vi "SHA-1 Test.vi"() -> ()   [LabVIEW 2021, in "WebSockets.lvlib" / "WebSocket.lvclass"]
doc: "WebSockets 2.0.1.40\nSam Sharp - MediaMongrels Ltd\nCopyright (c) 2019, MediaMongrels Ltd"
uses:
  WebSocket/WebSocket.lvclass
panel:
  out "SHA1 Data":u8[](array[numeric])=[0, 0, 0, 244, 146, 20, 24, 169, 106, 74, 162, 189, 106, 208, 220, 75, 21, 127, 121, 135] format="%.0x"
  in  "String":string
  # "SHA1(\"\")\n = da39a3ee 5e6b4b0d 3255bfef 95601890 afd80709"
  # "SHA1(\"The quick brown fox jumps over the lazy dog\") \n = 2fd4e1c6 7a2d28fc ed849ee1 bb76e739 1b93eb12"
  # "minor change - dog -> cog (notice large change, aka avalache effect, in digest)"
  # "SHA1(\"The quick brown fox jumps over the lazy cog\") \n = de9f2c7f d25e1b3a fad3e85a 0bd17d9b 100db4b3"
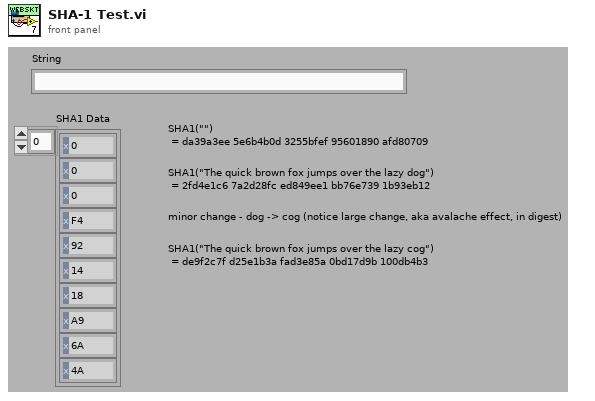
[diagram p1: front panel]
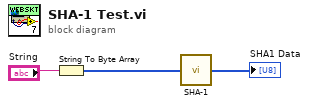
[diagram p0: block diagram]
diagram:
  n1 = String To Byte Array(string="String") -> (unsigned byte array=w2:u8[])
  n2 = call "SHA-1.vi"("Data"=w2) -> ("message-digest"=→"SHA1 Data":u8[])
